vi "Read Power Meter classes.vi"(11 "RF Power in":refnum<class "RF Power.lvclass">) -> (2 "Power Meter classes":refnum<class "Power Meter.lvclass">[](array[class]), 3 "RF Power out":refnum<class "RF Power.lvclass">)   [LabVIEW 2020, in "RF Power.lvclass"]
uses:
  RF Power.lvclass
  Instruments/Power Meter/Power Meter.lvclass
  RF Power.lvclass/RF Power.ctl
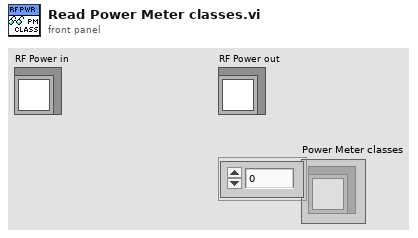
[diagram p1: front panel]
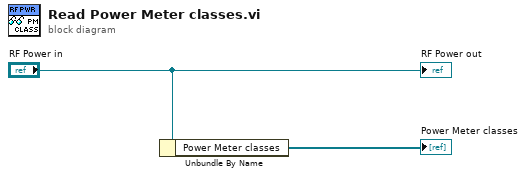
[diagram p0: block diagram]
diagram:
  n1 = Unbundle By Name("RF Power in") -> ("Power Meter classes"=→"Power Meter classes":refnum<class "Power Meter.lvclass">[])
  "RF Power out" <- "RF Power in"
